vi "XY Graph Add New Plot.vi"(0 "Multiplot XY Graph":T4, 1 "Scales (Default)":T2, 2 "Plot Interpolation (Previous Plot's Style)":T1=enum."Use Previous Plot's Style", 3 "Keep Existing Plots (T)":bool=TRUE, 7 "Plot Metadata":variant, 9 "New Plot Name in":string, 11 "error in (no error)":errorcluster, 13 "Plot Color (Default)":u32(colorbox)=15781887, 14 "Point Style (Dot)":T3=enum."Dot") -> (4 "XY Graph Caption":string, 8 "New Plot Index":i32, 10 "New Plot Name out":string, 15 "error out":errorcluster)   [LabVIEW 2021, in "XY Graph Add-Ons.lvlib"]
uses:
  XY Graph Add-Ons.lvlib
  XY Graph Refnum.ctl
  Plot Point Style.ctl
  Plot Scales.ctl
  LabVIEW Plot Interpolation.ctl
  Graphs.lvlib
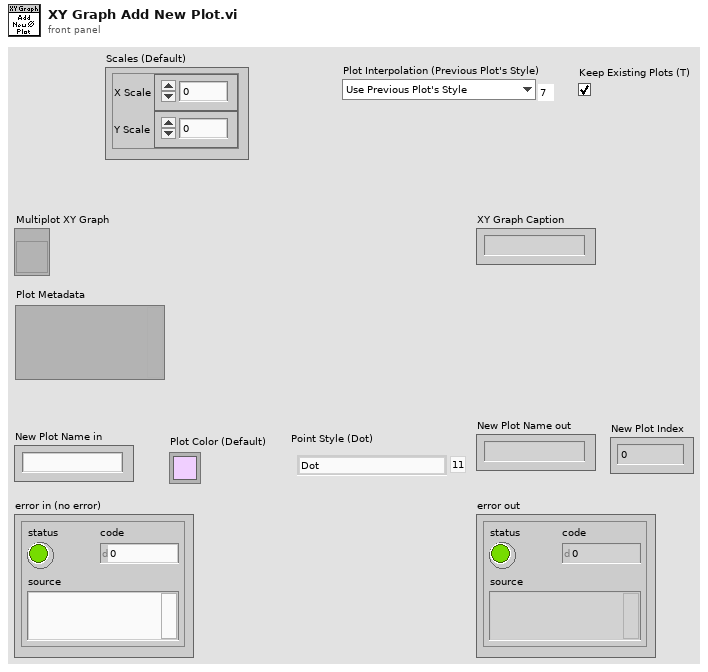
[diagram p1: front panel]
types:
  T1 = typedef "Graphs.lvlib/LabVIEW Plot Interpolation.ctl" = enum16{"Point (.)", "Stepwise Right (--.)", "Line + Point (\\. /)", "Stepwise Left (.--)", "Stepwise Centered (-.-)", "Stepwise Vertical (|.|)", "Line (-)", "Use Previous Plot's Style"}
  T2 = typedef "XY Graph Add-Ons.lvlib/Plot Scales.ctl" = cluster{"X Scale":u32, "Y Scale":u32}
  T3 = typedef "Graphs.lvlib/Plot Point Style.ctl" = enum16{"not defined", "None", "Empty Circle", "Filled Circle", "Thick Circle", "Dotted Circle", "Empty Square", "Filled Square", "Thick Square", "Dotted Square", "Small Filled Square", "Dot", "Cross", "Tiny Cross", "Large X", "Small x", "Diamond", "Small Empty Square"}
  T4 = typedef "XY Graph Add-Ons.lvlib/XY Graph Refnum.ctl" = refnum<vi>
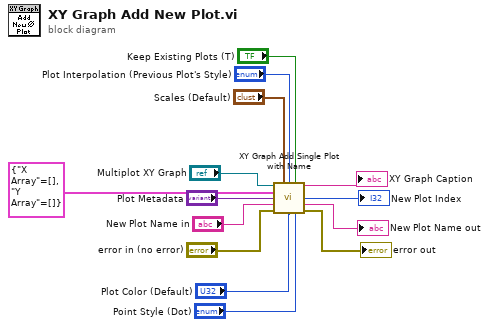
[diagram p0: block diagram]
diagram:
  n1 = call "XY Graph Add Single Plot with Name.vi"("XYGraph Ref in"="Multiplot XY Graph", "Scales (Default)"="Scales (Default)", "Plot Interpolation (Previous Plot's Style)"="Plot Interpolation (Previous Plot's Style)", "Keep Existing Plots (T)"="Keep Existing Plots (T)", "Plot"=cluster{"X Array":dbl[], "Y Array":dbl[]} {"X Array"=[], "Y Array"=[]} ("New Plot"), "Plot Metadata"="Plot Metadata", "Plot Name (\"Plot\")"="New Plot Name in", "error in (no error)"="error in (no error)", "Plot Color (Default)"="Plot Color (Default)", "Point Style (Dot)"="Point Style (Dot)") -> ("XY Graph Caption (or Label)"=→"XY Graph Caption":string, "Plot Index"=→"New Plot Index":i32, "Plot Name"=→"New Plot Name out":string, "error out"=→"error out":errorcluster)  [unwired: 2 in]
